vi "CreatePublicEvents.vi"(8 "error in (no error)":errorcluster, 11 "XYStage":refnum<class "XYStage.lvclass">) -> (0 "error out":errorcluster, 3 "XYStage out":refnum<class "XYStage.lvclass">)   [LabVIEW 2019, in "XYStage.lvclass"]
doc: "---------------------------------------------------------------\nJKI State Machine Objects™\nhttp://jki.net/state-machine-objects/\nCopyright (C) 2005-2015, JKI <info@jki.net>\nALL RIGHTS RESERVEDJKI State Machine Objects (SMO) 1.0.0.5\nJKI - JKI\nCopyright (c) 2016, JKI"
uses:
  XYStage.lvclass
  XYStage.lvclass/XYStage.ctl
  Typedefs/(real)Coords--Cluster.ctl
  Typedefs/PublicEvents--XYStage.UpdatedNamedPosition.ctl
  <vilib>/JKI/JKI SMO/SMO/SMO.lvclass
panel:
  # "For instructions on how to use the JKI State Machine Objects, examples and video tutorials, visit:\nhttp://jki.net/state-machine-objects/\n\nJKI State Machine Objects™\nhttp://jki.net/state-machine-objects/\nCopyright (C) 2005-2015, JKI <info@jki.net>\nALL RIGHTS RESERVED"
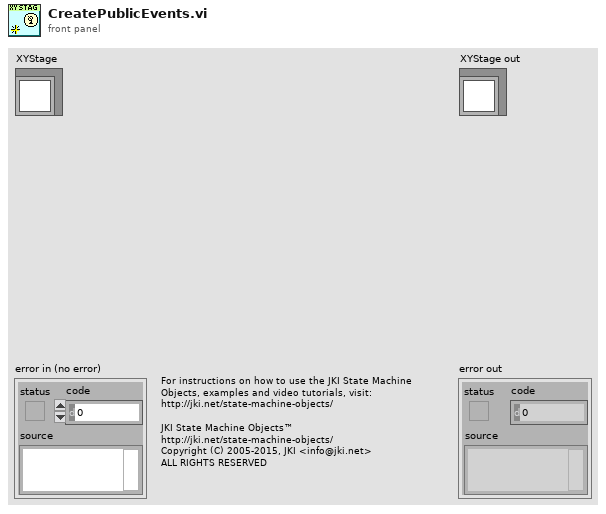
[diagram p1: front panel]
types:
  T1 = typedef "XYStage.lvclass/PrivateData--Ref.ctl" = refnum<data-value>
  T2 = typedef "XYStage.lvclass/PublicEvents--XYStage.UpdatedNamedPosition.ctl" = string
  T3 = typedef "XYStage.lvclass/(real)Coords--Cluster.ctl" = cluster{"X":dbl, "Y":dbl}
  T4 = typedef "XYStage.lvclass/PrivateData--Cluster.ctl" = cluster{"Dependencies":T5, "Public Events":T6, "Protected Events":T7, "Private Events":T8, "Configuration":T9, "Target":T10, "Move Parameters":T12}
  T5 = typedef "XYStage.lvclass/Dependencies--Cluster.ctl" = cluster{"Positions":refnum<class "SMO.Dictionary.Variant.lvclass">}
  T6 = typedef "XYStage.lvclass/PublicEvents--Cluster.ctl" = cluster{"MoveComplete":refnum<user-event>, "NewPosition":refnum<user-event>, "UpdatedNamedPosition":refnum<user-event>, "MoveStarted":refnum<user-event>}
  T7 = typedef "XYStage.lvclass/ProtectedEvents--Cluster.ctl" = cluster{"API_Template":refnum<user-event>}
  T8 = typedef "XYStage.lvclass/PrivateEvents--Cluster.ctl" = cluster{"MoveAbsolute":refnum<user-event>, "MoveRelative":refnum<user-event>, "MoveToNamedPosition":refnum<user-event>, "StorePosition":refnum<user-event>, "Home":refnum<user-event>}
  T9 = typedef "XYStage.lvclass/Configuration--Cluster.ctl" = cluster{"Real-World Units":string, "Counts per Unit":dbl}
  T10 = typedef "XYStage.lvclass/TargetPositions--Cluster.ctl" = cluster{"Coords":T3, "Counts":T11}
  T11 = typedef "XYStage.lvclass/(counts)Coords--Cluster.ctl" = cluster{"X":i32, "Y":i32}
  T12 = typedef "XYStage.lvclass/MoveParameters--Cluster.ctl" = cluster{"Velocity (units/s)":dbl, "Acceleration (units/s^2)":dbl}
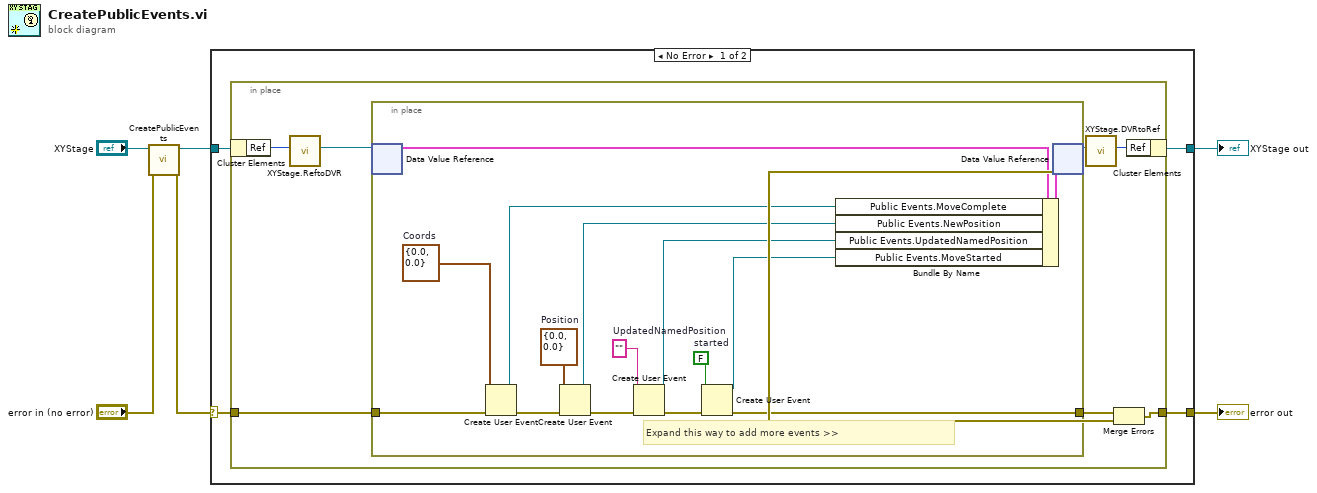
[diagram p0: block diagram]
diagram:
  n1 = call-parent "CreatePublicEvents.vi"("error in (no error)"="error in (no error)", "SMO"="XYStage") -> ("error out"=w1:errorcluster, "SMO out"=w3:refnum<class "XYStage.lvclass">)  [unwired: 8 in]
  n2 = case shown="No Error" w1 {
    selector: w1 -> [w8 w35]
    tunnel: [w7 w35] -> w5
    tunnel: [w9 w34] -> w6
    tunnel: w3 -> [w10 w34]
    frame No Error {
      n3 = in-place {
        in-place-border: w8 -> [w18]
        in-place-border: [w15] -> w7
        n4 = in-place-cluster #1(w10) -> ("Ref"=w14:u32)
        n5 = call "XYStage.ReftoDVR.vi"("Ref"=w14) -> ("Ref"=w13:T1)  [unwired: 10 in]
        n6 = in-place {
          in-place-border: w18 -> [w19]
          in-place-border: [w22] -> w17
          w21 = FALSE  # started
          w27 = T2 ""  # UpdatedNamedPosition
          w28 = T3 {"X"=0.0, "Y"=0.0}  # Position
          w31 = T3 {"X"=0.0, "Y"=0.0}  # Coords
          # "Expand this way to add more events >>"
          n7 = in-place-dvr #2(w13) -> (w25:T4)  [unwired: 1 out]
          n8 = Create User Event(user event datatype=w31, error in=w19) -> (user event=w32:refnum<user-event>, error out=w33:errorcluster)
          n9 = Create User Event(user event datatype=w28, error in=w33) -> (user event=w29:refnum<user-event>, error out=w30:errorcluster)
          n10 = Create User Event(user event datatype=w27, error in=w30) -> (user event=w26:refnum<user-event>, error out=w23:errorcluster)
          n11 = Create User Event(user event datatype=w21, error in=w23) -> (user event=w20:refnum<user-event>, error out=w22:errorcluster)
          n12 = Bundle By Name(cluster=w25, "Public Events.MoveComplete"=w32, "Public Events.NewPosition"=w29, "Public Events.UpdatedNamedPosition"=w26, "Public Events.MoveStarted"=w20) -> (w24:T4)
          n13 = in-place-dvr #2(w24) -> (w12:T1, w16:errorcluster)
        }
        n14 = call "XYStage.DVRtoRef.vi"("Ref"=w12) -> ("Ref"=w11:u32)  [unwired: 10 in]
        n15 = Merge Errors(w17, w16) -> (w15:errorcluster)
        n16 = in-place-cluster #1("Ref"=w11) -> (w9:refnum<class "XYStage.lvclass">)
      }
    }
    frame Error {
    }
  }
  "error out" <- w5
  "XYStage out" <- w6
